vi "rate safety.vi"(9 "Cutoff Rate":dbl=0.2, 10 "Desired Rate":dbl, 11 "Encoder Rate":dbl) -> (2 "Output Rate":dbl, 3 "Encoder Rate Out":dbl, 4 "No Rate Read":bool, 6 "Encoder Failure":bool)   [LabVIEW 2014]
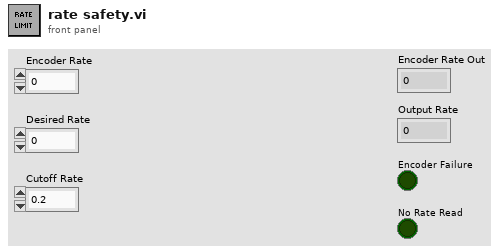
[diagram p1: front panel]
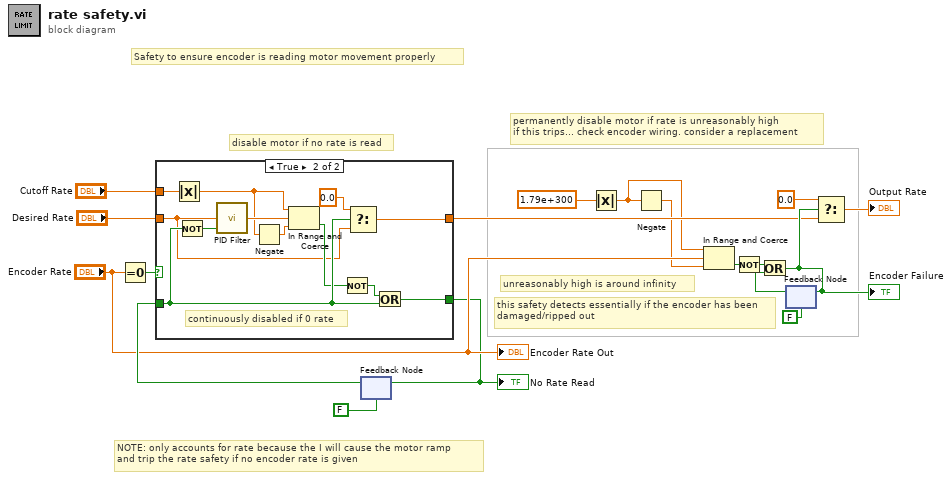
[diagram p0: block diagram]
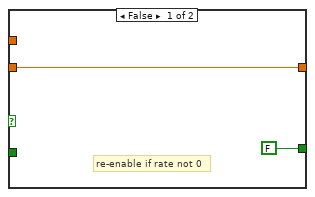
[diagram p2: hidden frame]
diagram:
  # "this safety detects essentially if the encoder has been\ndamaged/ripped out"
  # "unreasonably high is around infinity"
  # "permanently disable motor if rate is unreasonably high\nif this trips... check encoder wiring. consider a replacement"
  # "Safety to ensure encoder is reading motor movement properly"
  # "NOTE: only accounts for rate because the I will cause the motor ramp\nand trip the rate safety if no encoder rate is given"
  # "disable motor if no rate is read"
  n1 = Equal To 0?(x="Encoder Rate") -> (x = 0?=w17:bool)
  n2 = feedback #1(FALSE ("x > y?")) -> (w13:bool)
  n3 = case shown="True" w17 {
    tunnel: "Desired Rate" -> [w20 w22]
    tunnel: [w20 w31] -> w12
    tunnel: [FALSE w29] -> w9
    tunnel: w13 -> [_ w28]
    tunnel: "Cutoff Rate" -> [_ w26]
    frame False {
      # "re-enable if rate not 0"
    }
    frame True {
      # "continuously disabled if 0 rate"
      n4 = Absolute Value(x=w26) -> (abs(x)=w21:dbl)
      n5 = Not(x=w28) -> (.not. x?=w25:bool)
      n6 = call "PID Filter.vi"("reinitialize? (F)"=w25, "input"=w22) -> ("output"=w24:dbl)  [unwired: 3 in]
      n7 = Negate(x=w21) -> (-x=w27:dbl)
      n8 = In Range and Coerce(upper limit=w21, x=w24, lower limit=w27) -> (In Range?=w23:bool)  [unwired: 1 out]
      n9 = Not(x=w23) -> (.not. x?=w30:bool)
      n10 = Select(t=0.0, s=w28, f=w22) -> (s? t:f=w31:dbl)
      n11 = Or(x=w30, y=w28) -> (x .or. y?=w29:bool)
    }
  }
  "No Rate Read" <- w9
  n12 = feedback-in #1(w9) -> ()
  n13 = Absolute Value(x=1.79e+300 ("Max Rate")) -> (abs(x)=w1:dbl)
  n14 = Negate(x=w1) -> (-x=w3:dbl)
  n15 = In Range and Coerce(upper limit=w1, x="Encoder Rate", lower limit=w3) -> (In Range?=w5:bool)  [unwired: 1 out]
  n16 = Not(x=w5) -> (.not. x?=w4:bool)
  n17 = feedback #2(FALSE ("x > y?")) -> (w6:bool)
  n18 = Or(x=w4, y=w6) -> (x .or. y?=w16:bool)
  "Encoder Failure" <- w16
  n19 = feedback-in #2(w16) -> ()
  n20 = Select(t=0.0, s=w16, f=w12) -> (s? t:f=→"Output Rate":dbl)
  "Encoder Rate Out" <- "Encoder Rate"
